vi "PID Modified_Macro.vi"(7 "Diff Press Setpoint":dbl=40.0 format="%.2f", 8 "Supply Pressure":dbl, 9 "Tolerance":dbl=0.1 format="%.3f", 10 "Differential Pressure":dbl) -> (1 "In Range?":bool=TRUE, 3 "BP Output":dbl)   [LabVIEW 2018]
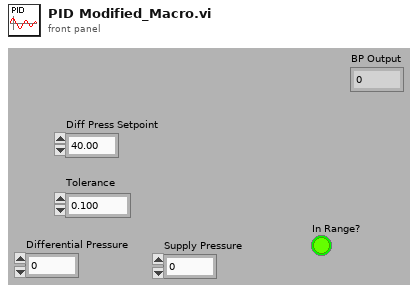
[diagram p1: front panel]
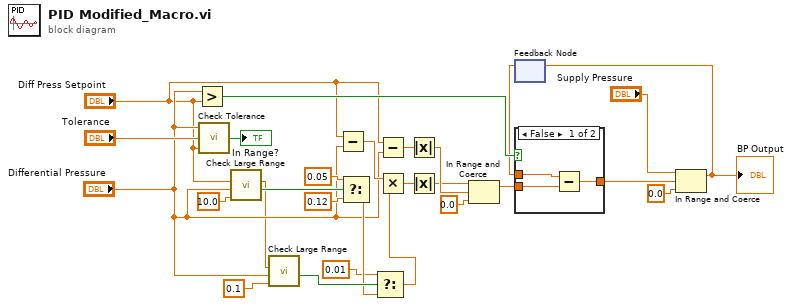
[diagram p0: block diagram]
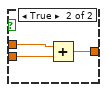
[diagram p2: hidden frame]
diagram:
  n1 = Greater?(x="Differential Pressure", y="Diff Press Setpoint") -> (0:w23:bool)
  n2 = call "Check Tolerance.vi"("setpoint"="Diff Press Setpoint", "Tolerance"="Tolerance", "Process variable"="Differential Pressure") -> ("Boolean"=→"In Range?":bool)
  n3 = call "Check Large Range.vi"("Tolerance"=10.0, "Differential Pressure"="Differential Pressure", "Diff Press Setpoint"="Diff Press Setpoint") -> ("In Range?"=w11:bool)  [unwired: 8 in]
  n4 = call "Check Large Range.vi"("Tolerance"=0.1, "Differential Pressure"="Differential Pressure", "Diff Press Setpoint"="Diff Press Setpoint") -> ("In Range?"=w6:bool)  [unwired: 8 in]
  n5 = Subtract(x="Diff Press Setpoint", y="Differential Pressure") -> (x-y=w15:dbl)
  n6 = Select(t=0.05, s=w11, f=0.12 ("Percent of Difference")) -> (s? t:f=w5:dbl)
  n7 = Select(t=0.01, s=w6, f=w5) -> (s? t:f=w4:dbl)
  n8 = Subtract(x="Diff Press Setpoint", y="Differential Pressure") -> (x-y=w24:dbl)
  n9 = Multiply(x=w15, y=w4) -> (x*y=w13:dbl)
  n10 = Absolute Value(x=w24) -> (abs(x)=w17:dbl)
  n11 = Absolute Value(x=w13) -> (abs(x)=w14:dbl)
  n12 = In Range and Coerce(upper limit=w14, x=w17, lower limit=0.0) -> (coerced(x)=w16:dbl)  [unwired: 1 out]
  n13 = feedback #1() -> (w22:dbl)  [unwired: 1 in]
  n14 = case shown="False" w23 {
    tunnel: w16 -> [w29 w32]
    tunnel: [w28 w31] -> w21
    tunnel: w22 -> [w27 w30]
    frame False {
      n15 = Subtract(x=w27, y=w29) -> (x-y=w28:dbl)
    }
    frame True {
      n16 = Add(x=w30, y=w32) -> (x+y=w31:dbl)
    }
  }
  n17 = In Range and Coerce(upper limit="Supply Pressure", x=w21, lower limit=0.0) -> (coerced(x)=w20:dbl)  [unwired: 1 out]
  "BP Output" <- w20
  n18 = feedback-in #1(w20) -> ()
